vi "ziSetValue.vi"   [LabVIEW 2009, in "Zurich Instruments LabOne.lvlib"]
doc: "This polymorphic vi sets values to nodes specified by <b>Path</b> to <b>Value</b>. More than one node can be set if a wildcard is used in the <b>Path</b>."
uses:
  <instrlib>/Zurich Instruments LabOne/Zurich Instruments LabOne.lvlib
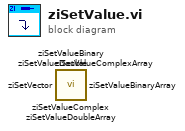
[diagram p0: block diagram]
diagram:
  n1 = call <instrlib>:"ziSetValueComplex.vi"() -> ()  [unwired: 5 in, 2 out]
  n2 = call <instrlib>:"ziSetValueComplexArray.vi"() -> ()  [unwired: 5 in, 2 out]
  n3 = call <instrlib>:"ziSetVector.vi"() -> ()  [unwired: 4 in, 3 out]
  n4 = call <instrlib>:"ziSetValueBinaryArray.vi"() -> ()  [unwired: 5 in, 2 out]
  n5 = call <instrlib>:"ziSetValueDoubleArray.vi"() -> ()  [unwired: 5 in, 2 out]
  n6 = call <instrlib>:"ziSetValueBinary.vi"() -> ()  [unwired: 5 in, 2 out]
  n7 = call <instrlib>:"ziSetValueDouble.vi"() -> ()  [unwired: 5 in, 2 out]
